vi "CreatePaths.vi"() -> (0 "ConfigFilesPath":path, 1 "LibPath":path)   [LabVIEW 2018, in "Config.lvlib"]
uses:
  Config/Config.lvlib
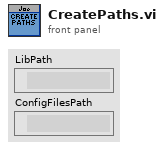
[diagram p1: front panel]
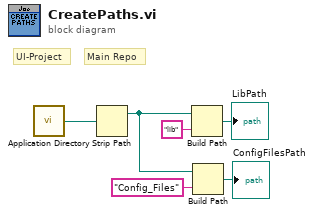
[diagram p0: block diagram]
diagram:
  # "UI-Project"
  # "Main Repo"
  n1 = call <vilib>:"Application Directory.vi"() -> ("Application Directory"=w6:path)
  n2 = Strip Path(path=w6) -> (stripped path=w3:path)  [unwired: 1 out]
  n3 = Build Path(base path=w3, name or relative path="lib") -> (appended path=→"LibPath":path)
  n4 = Build Path(base path=w3, name or relative path="Config_Files") -> (appended path=→"ConfigFilesPath":path)
